vi "Set Verbose Linker Errors.vi"(8 "error in (no error)":errorcluster, 10 "Verbose Linker Errors? (true)":bool=TRUE, 11 "SDIST in":refnum<class "NI_AB_API_DSDIST.lvclass">) -> (0 "error out":errorcluster, 3 "SDIST out":refnum<class "NI_AB_API_DSDIST.lvclass">)   [LabVIEW 2020, in "NI_AB_API_DSDIST.lvclass"]
uses:
  <vilib>/AppBuilder/AB_API/DSDIST/NI_AB_API_DSDIST.lvclass
  <vilib>/AppBuilder/AB_API/SDIST/NI_AB_API_SDIST.lvclass
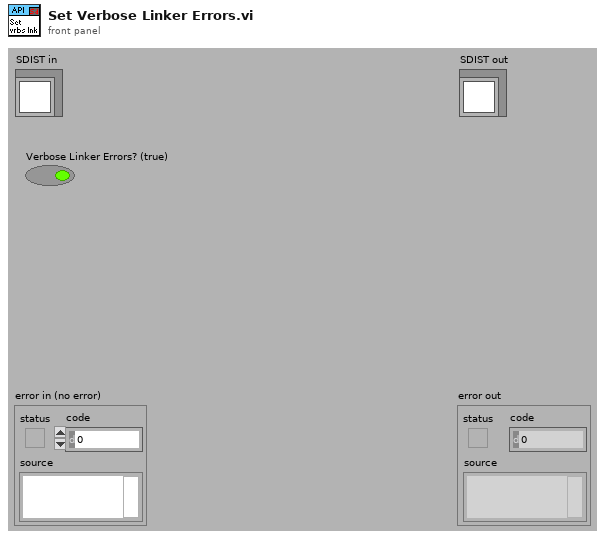
[diagram p1: front panel]
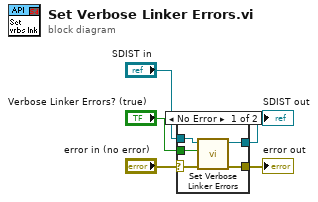
[diagram p0: block diagram]
diagram:
  n1 = case shown="No Error" "error in (no error)" {
    selector: "error in (no error)" -> [w7 w12]
    tunnel: [w8 w12] -> w4
    tunnel: [w9 w11] -> w2
    tunnel: "SDIST in" -> [w10 w11]
    tunnel: "Verbose Linker Errors? (true)" -> [w6 _]
    frame No Error {
      n2 = call-parent "Set Verbose Linker Errors.vi"("error in (no error)"=w7, "Verbose Linker Errors? (true)"=w6, "SDIST in"=w10) -> ("error out"=w8:errorcluster, "SDIST out"=w9:refnum<class "NI_AB_API_DSDIST.lvclass">)  [unwired: 7 in]
    }
    frame Error {
    }
  }
  "error out" <- w4
  "SDIST out" <- w2
